vi "Update Table.vi"(5 "Table map":refnum<vi>, 7 "Limit (10k)":i32=10000 format="%.0p", 8 "error in":errorcluster, 10 "New Data in":string[][](array[string]), 11 "Table Data in":string[][](array[string])) -> (0 "error out":errorcluster, 3 "Table Data out":string[][](array[string]))   [LabVIEW 2025, in "CAN-LIN Raw Bus Capture UI.lvlib"]
doc: "Update the Table with the new data. Only overwrite if new data is avaliable."
uses:
  CAN-LIN Raw Bus Capture UI.lvlib
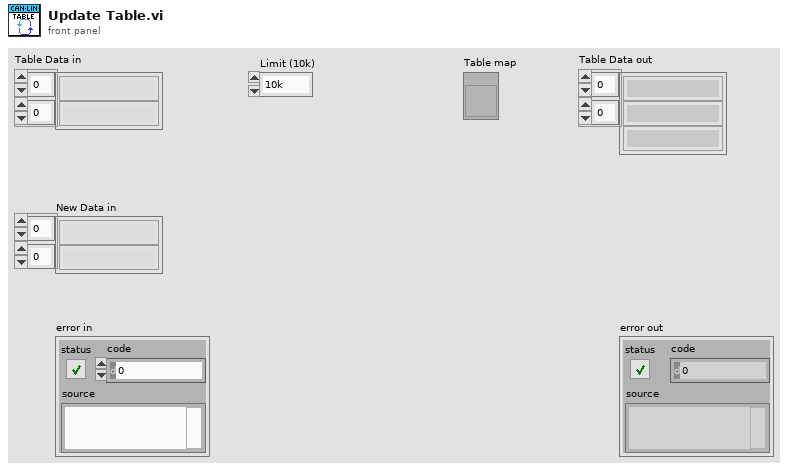
[diagram p1: front panel]
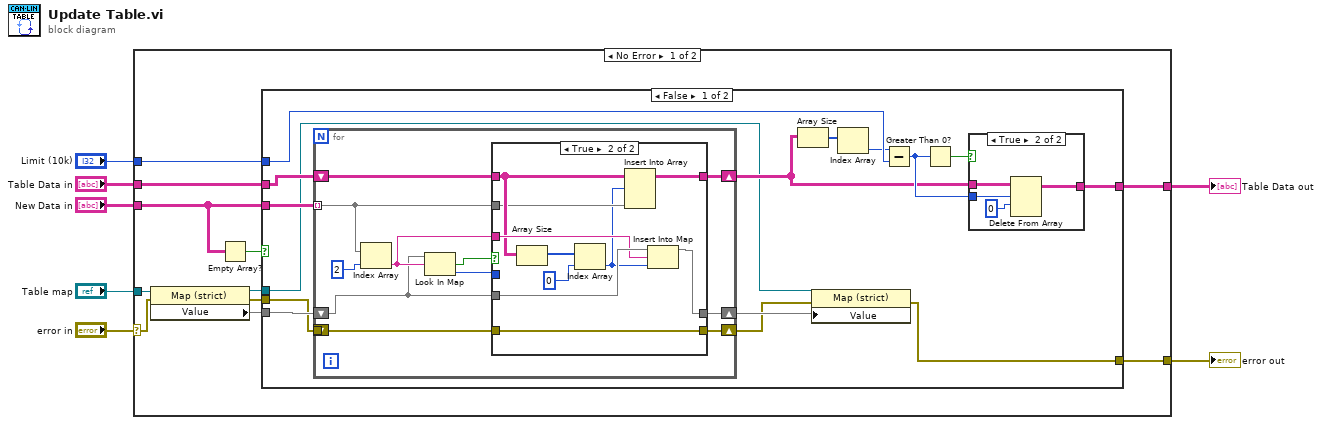
[diagram p0: block diagram]
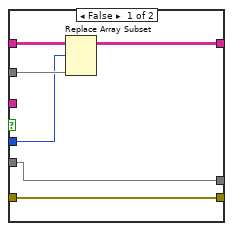
[diagram p2: hidden frame]
diagram:
  n1 = case shown="No Error" "error in" {
    selector: "error in" -> [w8 w69]
    tunnel: "New Data in" -> [w16 _]
    tunnel: [w18 w69] -> w5
    tunnel: "Limit (10k)" -> [w14 _]
    tunnel: "Table Data in" -> [w13 w68]
    tunnel: [w15 w68] -> w2
    tunnel: "Table map" -> [w9 _]
    frame No Error {
      n2 = property class="Map (strict)"(reference=w9, error in=w8) -> (reference out=w12:refnum<vi>, error out=w11:errorcluster, "Value"=w10:map{string, i32})
      n3 = Empty Array?(array=w16) -> (empty?=w17:bool)
      n4 = case shown="False" w17 {
        tunnel: w16 -> [w27 _]
        tunnel: [w19 w66] -> w18
        tunnel: w14 -> [w33 _]
        tunnel: w13 -> [w25 w67]
        tunnel: [w32 w67] -> w15
        tunnel: w12 -> [w21 _]
        tunnel: w11 -> [w23 w66]
        tunnel: w10 -> [w24 _]
        frame False {
          n5 = for {
            tunnel: w27 -> [w42] mode=indexing
            shift-right: [w39] -> w26
            shift-left: w25 -> [w43]
            shift-right: [w37] -> w20
            shift-left: w23 -> [w35]
            tunnel: [w35] -> _
            shift-right: [w34] -> w22
            shift-left: w24 -> [w36]
            n6 = Index Array(array=w42, index=2) -> (element=w40:string)
            n7 = Look In Map(map=w36, key=w40) -> (key not found?=w41:bool, value=w38:i32)  [unwired: 1 in]
            n8 = case shown="True" w41 {
              tunnel: w43 -> [w50 w56]
              tunnel: [w47 w54] -> w39
              tunnel: w42 -> [w49 w55]
              tunnel: w38 -> [w48 _]
              tunnel: w36 -> [w45 w60]
              tunnel: w40 -> [_ w57]
              tunnel: w35 -> [w46 w51]
              tunnel: [w46 w51] -> w37
              tunnel: [w45 w52] -> w34
              frame False {
                n9 = Replace Array Subset(array=w50, new element=w49, index (row)=w48) -> (w47:string[][])  [unwired: 1 in]
              }
              frame True {
                n10 = Array Size(array=w56) -> (size(s)=w59:i32[])
                n11 = Index Array(array=w59, index=0) -> (element=w53:i32)
                n12 = Insert Into Array(array=w56, index (row)=w53, new element=w55) -> (w54:string[][])  [unwired: 1 in]
                n13 = Insert Into Map(map in=w60, key=w57, value=w53) -> (map out=w52:map{string, i32})  [unwired: 2 out]
              }
            }
          }
          n14 = Array Size(array=w26) -> (size(s)=w31:i32[])
          n15 = property class="Map (strict)"(reference=w21, error in=w20, "Value"=w22) -> (error out=w19:errorcluster)  [unwired: 1 out]
          n16 = Index Array(array=w31) -> (element=w30:i32)  [unwired: 1 in]
          n17 = Subtract(x=w30, y=w33) -> (x-y=w28:i32)
          n18 = Greater Than 0?(x=w28) -> (x > 0?=w29:bool)
          n19 = case shown="True" w29 {
            tunnel: w26 -> [w61 w65]
            tunnel: [w61 w64] -> w32
            tunnel: w28 -> [_ w63]
            frame False {
            }
            frame True {
              n20 = Delete From Array(array=w65, length=w63, index (row)=0) -> (array with subset deleted=w64:string[][])  [unwired: 1 in, 1 out]
            }
          }
        }
        frame True {
        }
      }
    }
    frame Error {
    }
  }
  "error out" <- w5
  "Table Data out" <- w2
